vi "data_distributor.vi"(0 "Analog Data Array":T1[](array[typedef]), 7 "Refnums of Controls":T2[](array[typedef]), 9 "Indicies":T3[](array[typedef]), 11 "error in":errorcluster) -> (15 "error out":errorcluster)   [LabVIEW 2017]
uses:
  Utility Sub VIs/pressure_temp_mixture.ctl
  Utility Sub VIs/pulse_generator_data_charts.ctl
  Utility Sub VIs/pulse_generator_data.ctl
  Utility Sub VIs/diode_charts.ctl
  index_array_cluster.ctl
  refnum_array_cluster.ctl
  Utility Sub VIs/valve_pid_control.ctl
  Box/Annular Flow/Jason/LabVIEW 2017/Input Channel Lists/analog_data.ctl
panel:
  in  "PID Refnum":refnum<vi>
  in  "Diode ChartsRefnum":refnum<vi>
  in  "Measurements Data Refnum":refnum<vi>
  in  "PG Charts Refnum":refnum<vi>
  in  "Pressure/Temperature/Mixture Properties Refnum":refnum<vi>
  # "Pulse Gen"
  # "Test Section"
  # "Saturation\nPressure [Pa]"
  # "Saturation\nTemperature [C]"
  # "Pressure [Pa]"
  # "Temperature [C]"
  # "Liquid Tank"
  # "Separator"
  # "Liquid Inlet"
  # "Vapor Tank"
  # "Vapor Inlet"
  # "Test Section"
  # "Upper Dev Section"
  # "Lower Dev Section"
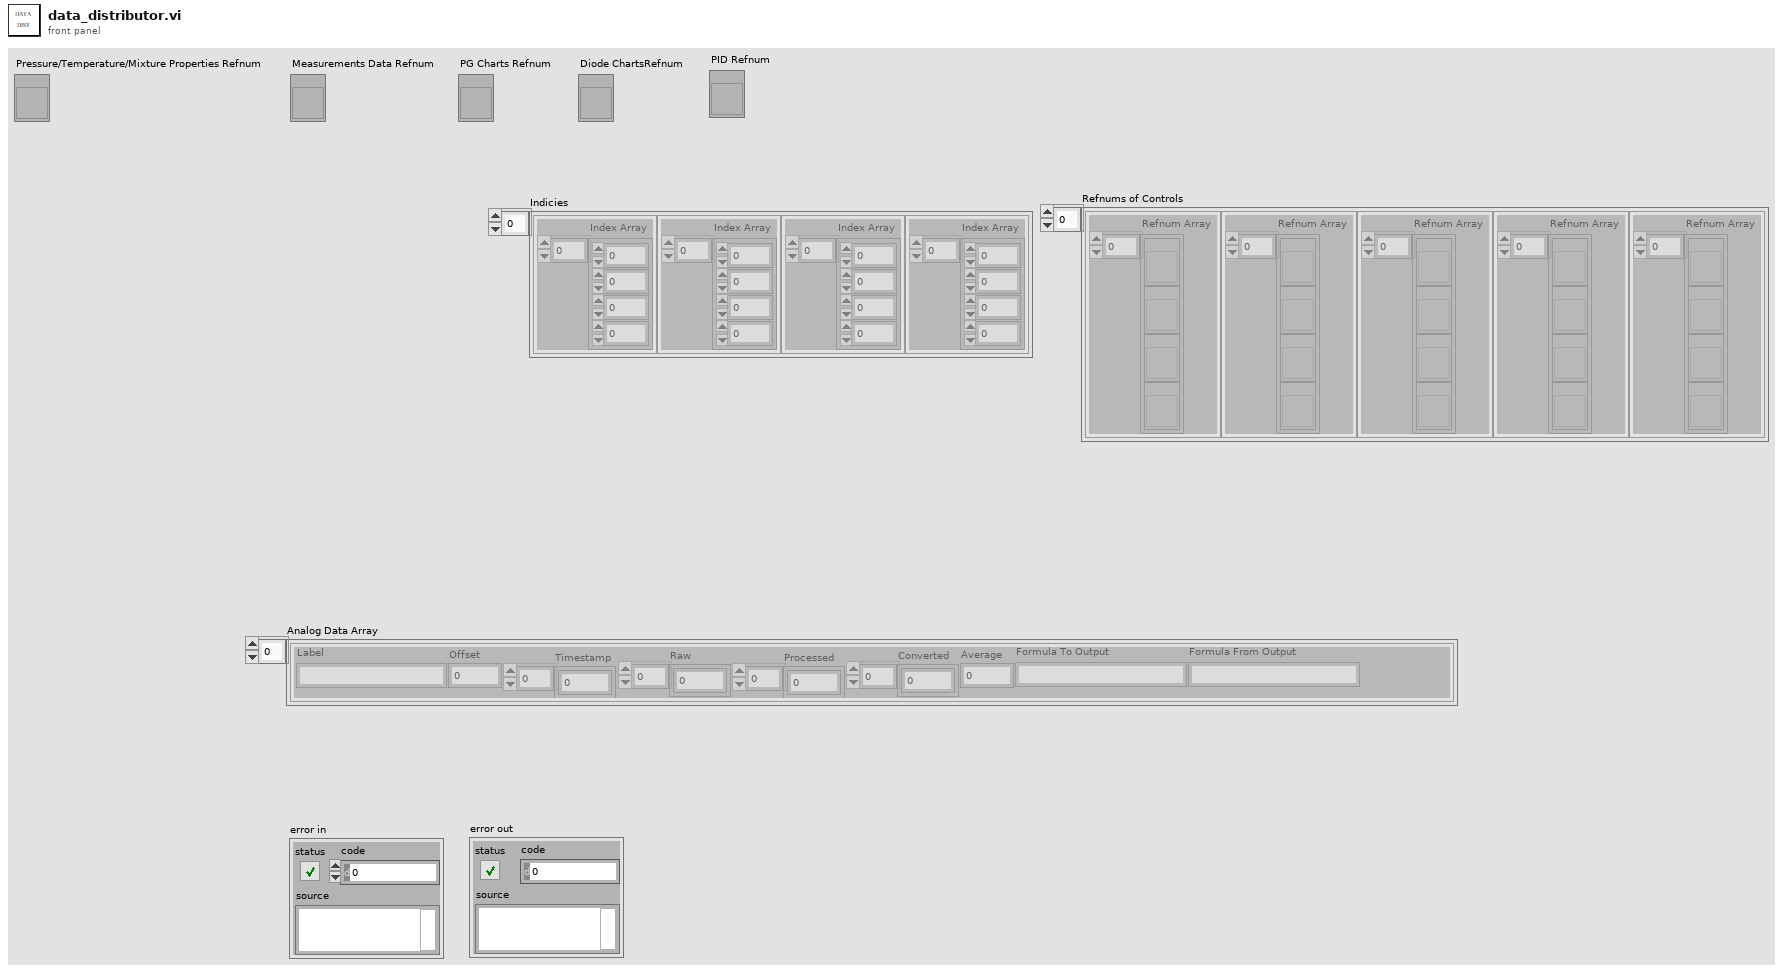
[diagram p1: front panel]
types:
  T1 = typedef "analog_data.ctl" = cluster{"Label":string, "Offset":dbl, "Timestamp":dbl[], "Raw":dbl[], "Processed":dbl[], "Converted":dbl[], "Average":dbl, "Formula To Output":string, "Formula From Output":string}
  T2 = typedef "refnum_array_cluster.ctl" = cluster{"Refnum Array":refnum<vi>[]}
  T3 = typedef "index_array_cluster.ctl" = cluster{"Index Array":i32[]}
  T4 = typedef "pressure_temp_mixture.ctl" = cluster{"Line Densities\n[g/cm^3]":cluster{"Vapor Line":dbl, "Liquid Line":dbl}, "Mixture Properties":cluster{"Enthalpy":dbl, "Quality [-]":dbl}, "Component PTs":cluster{"Liquid Tank P":dbl, "Liquid Tank T":dbl, "Liquid Tank Sat P":dbl, "Liquid Tank Sat T":dbl, "Separator P":dbl, "Separator T":dbl, "Separator Sat P":dbl, "Separator Sat T":dbl, "Liquid Inlet P":dbl, "Liquid Inlet T":dbl, "Liquid Inlet Sat P":dbl, "Liquid Inlet Sat T":dbl, "Vapor Tank P":dbl, "Vapor Tank T":dbl, "Vapor Tank Sat P":dbl, "Vapor Tank Sat T":dbl, "Vapor Inlet P":dbl, "Vapor Inlet T":dbl, "Vapor Inlet Sat P":dbl, "Vapor Inlet Sat T":dbl, "Test Section P":dbl, "Test Section T":dbl, "Test Section Sat P":dbl, "Test Section Sat T":dbl, "Upper Dev Section P":dbl, "Upper Dev Section T":dbl, "Upper Dev Section Sat P":dbl, "Upper Dev Section Sat T":dbl, "Lower Dev Section P":dbl, "Lower Dev Section T":dbl, "Lower Dev Section Sat P":dbl, "Lower Dev Section Sat T":dbl}, "Ambient Pressure [Pa]":dbl, "Mixing Tee":cluster{"Mixing Tee dP":dbl, "PG inlet-Mixing Tee Abs Pressure":dbl, "PG inlet-Mixing Tee Temperature":dbl}}
  T5 = cluster{"[0]":dbl, "[1]":dbl, "[2]":dbl, "[3]":dbl, "[4]":dbl, "[5]":dbl, "[6]":dbl, "[7]":dbl, "[8]":dbl, "[9]":dbl, "[10]":dbl, "[11]":dbl, "[12]":dbl, "[13]":dbl, "[14]":dbl, "[15]":dbl, "[16]":dbl, "[17]":dbl, "[18]":dbl, "[19]":dbl, "[20]":dbl, "[21]":dbl, "[22]":dbl, "[23]":dbl, "[24]":dbl, "[25]":dbl, "[26]":dbl, "[27]":dbl, "[28]":dbl, "[29]":dbl, "[30]":dbl, "[31]":dbl}
  T6 = cluster{"Mass Flow Rate [g/s]":dbl, "Mass Flow Rate [g/s]":dbl}
  T7 = cluster{"[0]":dbl, "[1]":dbl, "[2]":dbl, "[3]":dbl, "[4]":dbl, "[5]":dbl, "[6]":dbl, "[7]":dbl, "[8]":dbl, "[9]":dbl, "[10]":dbl, "[11]":dbl, "[12]":dbl, "[13]":dbl, "[14]":dbl, "[15]":dbl}
  T8 = typedef "valve_pid_control.ctl" = cluster{"proportional gain (Kc)":dbl, "integral time (Ti, min)":dbl, "derivative time (Td, min)":dbl, "Valve Voltage [V]":dbl, "Min % Open":dbl, "Max % Open":dbl, "Reinitialize?":bool, "Valve On/Off":bool, "Mode":bool, "Full Flow Rate":dbl, "Flow Set Point [g/s]":dbl, "AutoTune":bool, "Flow":cluster{"Flow rate [g/s]":dbl, "Line Density [g/cm^3]":dbl}}
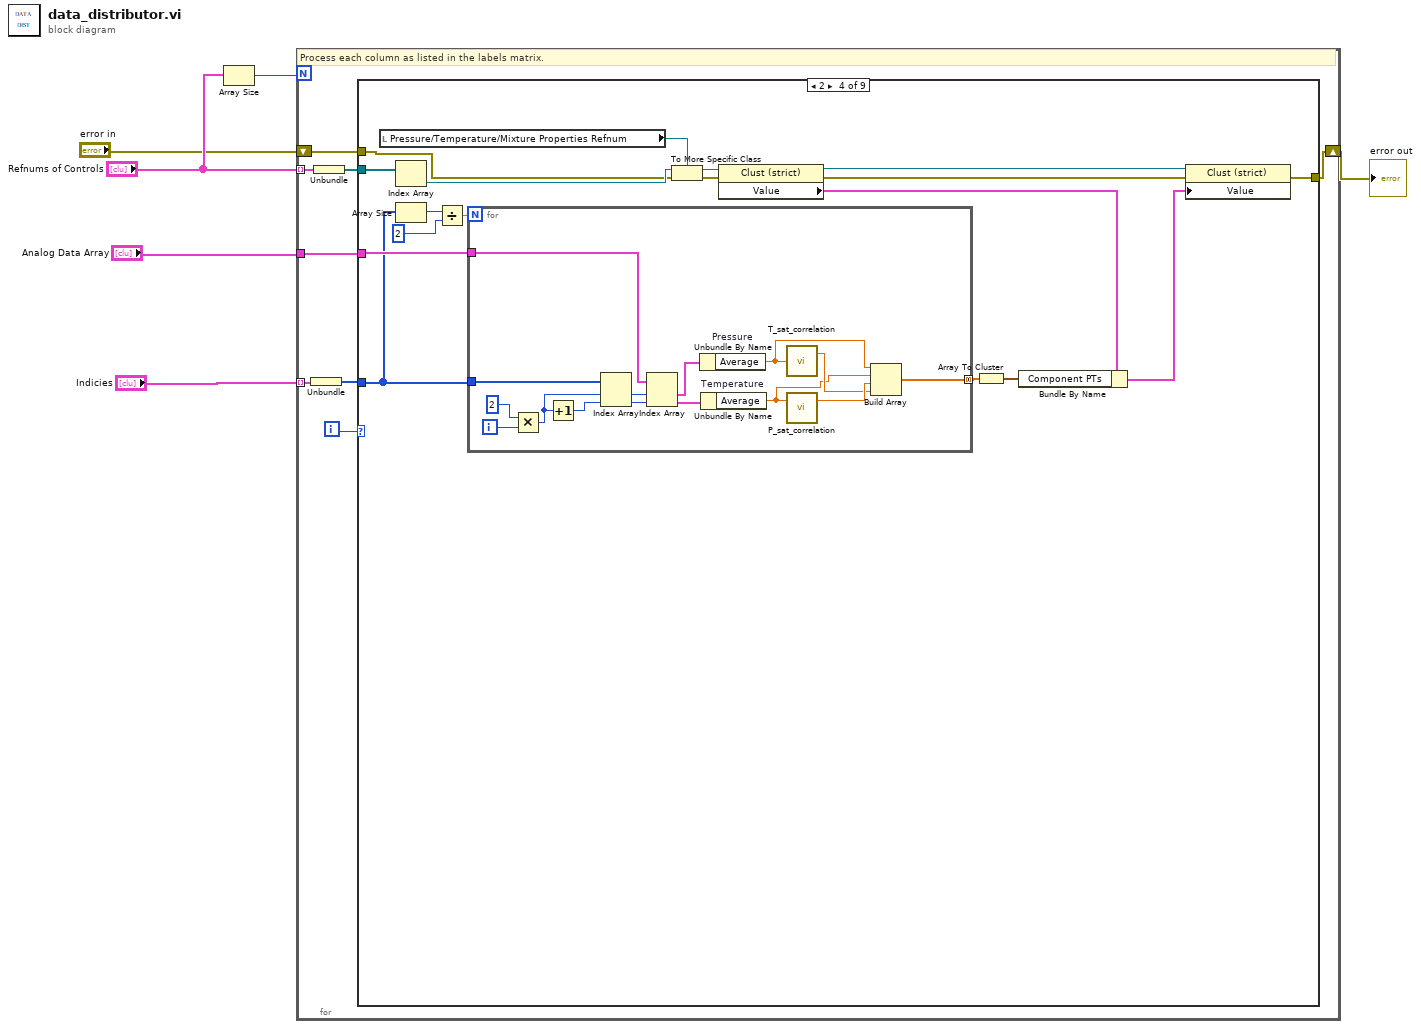
[diagram p0: block diagram]
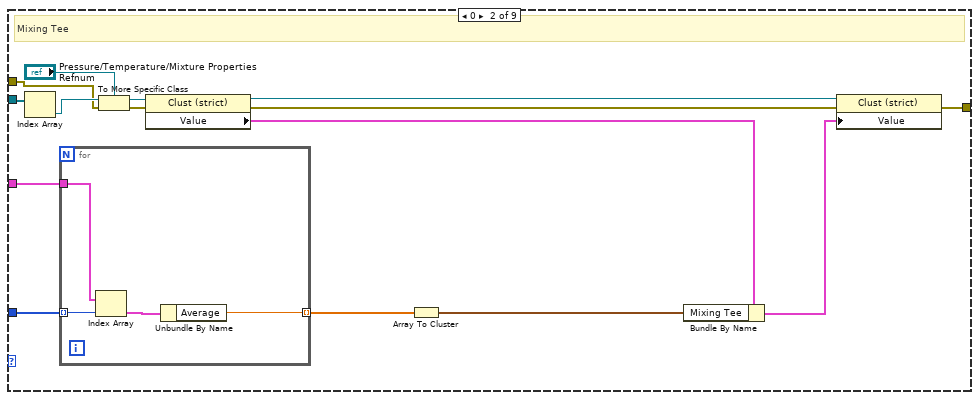
[diagram p3: hidden frame]
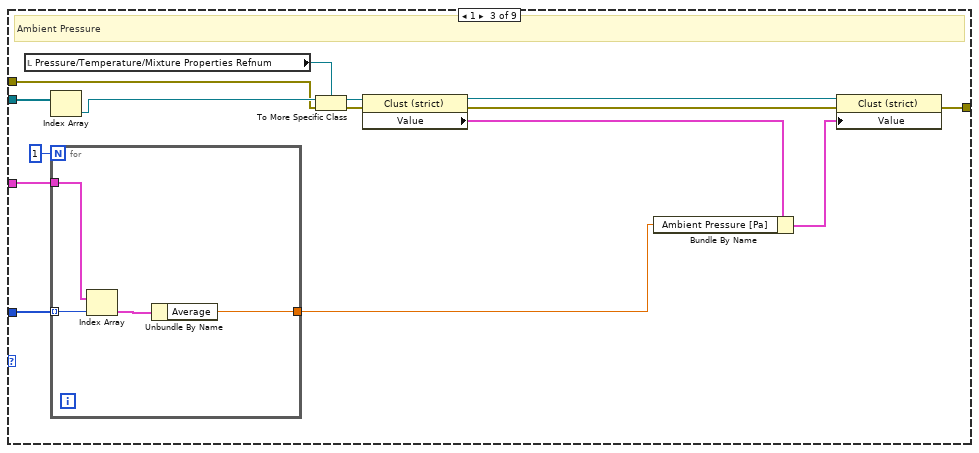
[diagram p4: hidden frame]
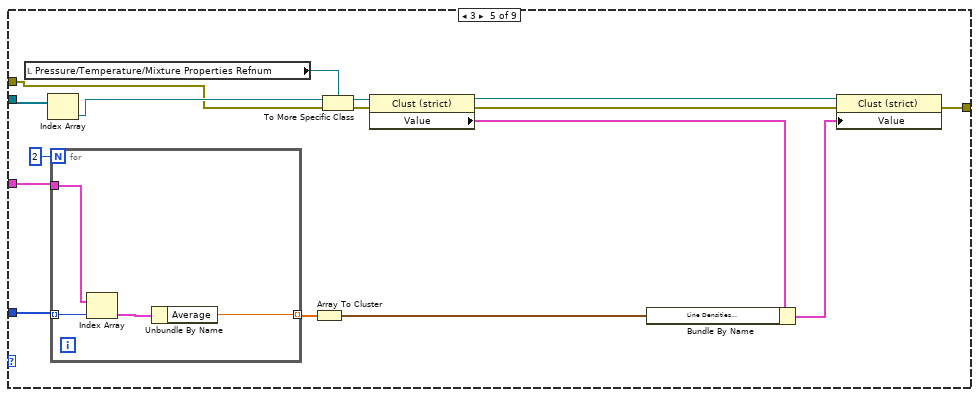
[diagram p5: hidden frame]
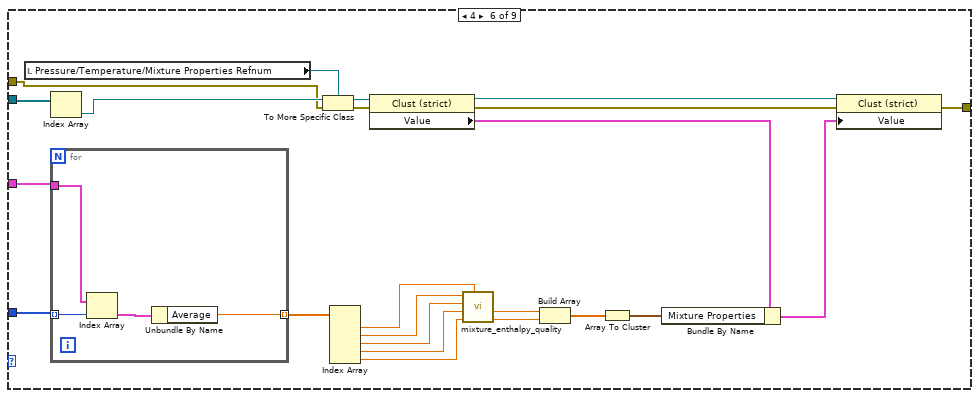
[diagram p6: hidden frame]
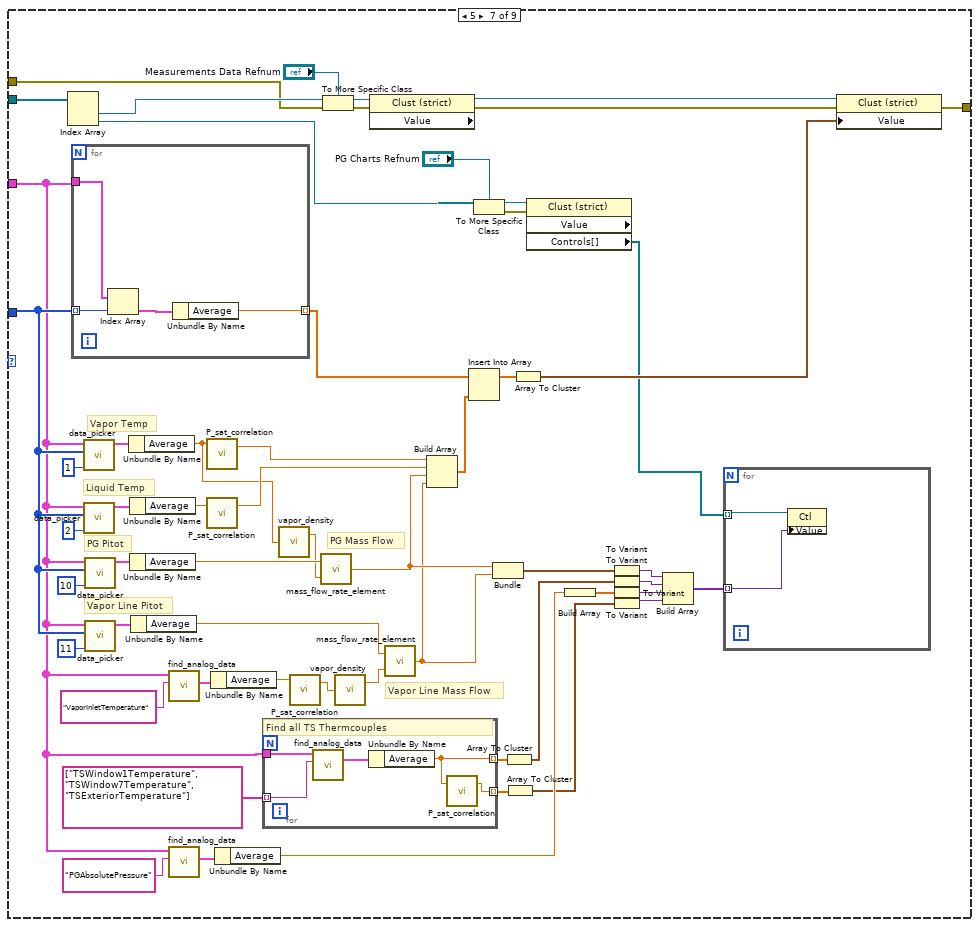
[diagram p7: hidden frame]
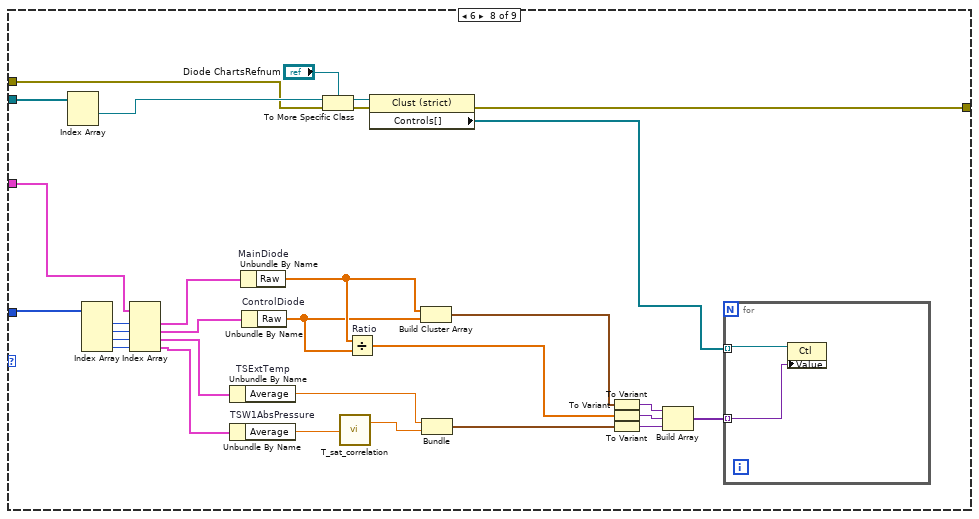
[diagram p8: hidden frame]
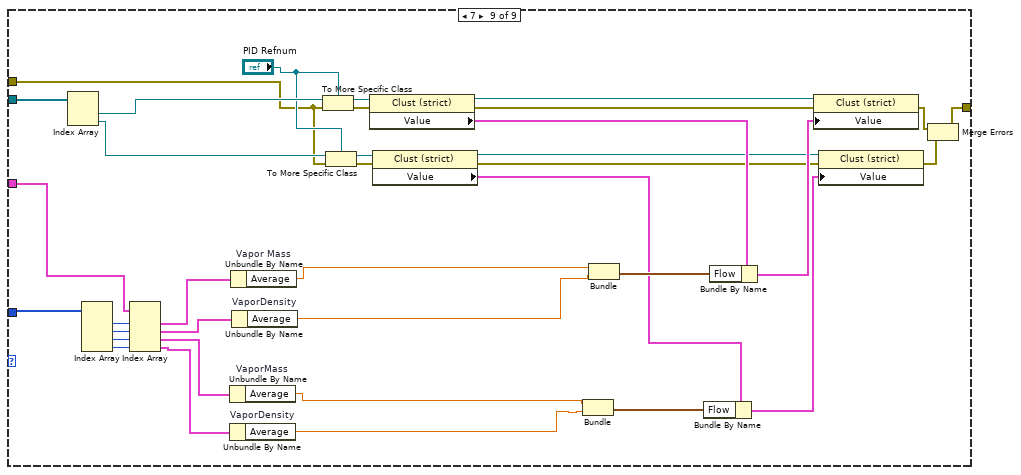
[diagram p9: hidden frame]
diagram:
  n1 = Array Size(array="Refnums of Controls") -> (size(s)=w3:i32)
  n2 = for {
    N: w3 -> [_]
    tunnel: "Analog Data Array" -> [w13]
    tunnel: "Indicies" -> [w10] mode=indexing
    tunnel: "Refnums of Controls" -> [w12] mode=indexing
    shift-right: [w7] -> w5
    shift-left: "error in" -> [w8]
    i -> [w14]
    # "Process each column as listed in the labels matrix."
    n3 = Unbundle(w10) -> ("Index Array"=w9:i32[])
    n4 = Unbundle(w12) -> ("Refnum Array"=w11:refnum<vi>[])
    n5 = case shown="2" w14 {
      tunnel: w9 -> [_ w23 w42 w63 w94 w121 w177 w221 w265]
      tunnel: w11 -> [_ w16 w38 w57 w90 w110 w147 w227 w266]
      tunnel: w13 -> [_ w22 w43 w64 w95 w122 w152 w219 w263]
      tunnel: w8 -> [w15 w18 w36 w55 w88 w108 w136 w203 w251]
      tunnel: [w15 w17 w35 w54 w87 w107 w135 w202 w234] -> w7
      frame Default {
      }
      frame 0 {
        # "Mixing Tee"
        n6 = Index Array(array=w16) -> (element=w19:refnum<vi>)  [unwired: 1 in]
        n7 = for {
          tunnel: w23 -> [w34] mode=indexing
          tunnel: w22 -> [w33]
          tunnel: [w31] -> w21 mode=indexing
          n8 = Index Array(array=w33, index=w34) -> (element=w32:T1)
          n9 = Unbundle By Name(w32) -> ("Average"=w31:dbl)
        }
        n10 = To More Specific Class(target class="Pressure/Temperature/Mixture Properties Refnum", reference=w19, error in=w18) -> (specific class reference=w29:refnum<vi>, error out=w28:errorcluster)
        n11 = property class="Clust (strict)"(reference=w29, error in=w28) -> (reference out=w24:refnum<vi>, error out=w25:errorcluster, "Value"=w27:T4)
        n12 = Array To Cluster(array=w21) -> (cluster=w20:cluster{"[0]":dbl, "[1]":dbl, "[2]":dbl})
        n13 = Bundle By Name(cluster=w27, "Mixing Tee"=w20) -> (w26:T4)
        n14 = property class="Clust (strict)"(reference=w24, error in=w25, "Value"=w26) -> (error out=w17:errorcluster)  [unwired: 1 out]
      }
      frame 1 {
        # "Ambient Pressure"
        n15 = local read "Pressure/Temperature/Mixture Properties Refnum"() -> (w40:refnum<vi>)
        n16 = Index Array(array=w38) -> (element=w37:refnum<vi>)  [unwired: 1 in]
        n17 = for {
          N: 1 -> [_]
          tunnel: w42 -> [w53] mode=indexing
          tunnel: w43 -> [w52]
          tunnel: [w50] -> w41
          n18 = Index Array(array=w52, index=w53) -> (element=w51:T1)
          n19 = Unbundle By Name(w51) -> ("Average"=w50:dbl)
        }
        n20 = To More Specific Class(target class=w40, reference=w37, error in=w36) -> (specific class reference=w49:refnum<vi>, error out=w48:errorcluster)
        n21 = property class="Clust (strict)"(reference=w49, error in=w48) -> (reference out=w44:refnum<vi>, error out=w45:errorcluster, "Value"=w47:T4)
        n22 = Bundle By Name(cluster=w47, "Ambient Pressure [Pa]"=w41) -> (w46:T4)
        n23 = property class="Clust (strict)"(reference=w44, error in=w45, "Value"=w46) -> (error out=w35:errorcluster)  [unwired: 1 out]
      }
      frame 2 {
        n24 = local read "Pressure/Temperature/Mixture Properties Refnum"() -> (w65:refnum<vi>)
        n25 = Index Array(array=w57) -> (element=w56:refnum<vi>)  [unwired: 1 in]
        n26 = Array Size(array=w63) -> (size(s)=w61:i32)
        n27 = Divide(x=w61, y=2) -> (x/y=w62:dbl)
        n28 = for {
          N: w62 -> [_]
          tunnel: w63 -> [w82]
          tunnel: w64 -> [w86]
          tunnel: [w72] -> w59 mode=concatenating
          i -> [w84]
          n29 = Multiply(x=2, y=w84) -> (x*y=w80:i32)
          n30 = Increment(x=w80) -> (x+1=w81:i32)
          n31 = Index Array(array=w82, index #1=w80, index #2=w81) -> (element #1=w79:i32, element #2=w78:i32)
          n32 = Index Array(array=w86, index #1=w79, index #2=w78) -> (element #1=w85:T1, element #2=w77:T1)
          n33 = Unbundle By Name "Pressure"(w85) -> ("Average"=w74:dbl)
          n34 = Unbundle By Name "Temperature"(w77) -> ("Average"=w73:dbl)
          n35 = call "T_sat_correlation.vi"("P [Pa]"=w74) -> ("T Sat [C]"=w75:dbl)  [unwired: 1 out]
          n36 = call "P_sat_correlation.vi"("Temperature[C]"=w73) -> ("P Sat[Pa]"=w76:dbl)  [unwired: 1 in, 1 out]
          n37 = Build Array(w74, w73, w76, w75) -> (w72:dbl[])
        }
        n38 = To More Specific Class(target class=w65, reference=w56, error in=w55) -> (specific class reference=w71:refnum<vi>, error out=w70:errorcluster)
        n39 = property class="Clust (strict)"(reference=w71, error in=w70) -> (reference out=w66:refnum<vi>, error out=w67:errorcluster, "Value"=w69:T4)
        n40 = Array To Cluster(array=w59) -> (cluster=w58:T5)
        n41 = Bundle By Name(cluster=w69, "Component PTs"=w58) -> (w68:T4)
        n42 = property class="Clust (strict)"(reference=w66, error in=w67, "Value"=w68) -> (error out=w54:errorcluster)  [unwired: 1 out]
      }
      frame 3 {
        n43 = local read "Pressure/Temperature/Mixture Properties Refnum"() -> (w96:refnum<vi>)
        n44 = Index Array(array=w90) -> (element=w89:refnum<vi>)  [unwired: 1 in]
        n45 = for {
          N: 2 -> [_]
          tunnel: w94 -> [w106] mode=indexing
          tunnel: w95 -> [w105]
          tunnel: [w103] -> w93 mode=indexing
          n46 = Index Array(array=w105, index=w106) -> (element=w104:T1)
          n47 = Unbundle By Name(w104) -> ("Average"=w103:dbl)
        }
        n48 = Array To Cluster(array=w93) -> (cluster=w92:cluster{"[0]":dbl, "[1]":dbl})
        n49 = To More Specific Class(target class=w96, reference=w89, error in=w88) -> (specific class reference=w102:refnum<vi>, error out=w101:errorcluster)
        n50 = property class="Clust (strict)"(reference=w102, error in=w101) -> (reference out=w97:refnum<vi>, error out=w98:errorcluster, "Value"=w100:T4)
        n51 = Bundle By Name(cluster=w100, "Line Densities\n[g/cm^3]"=w92) -> (w99:T4)
        n52 = property class="Clust (strict)"(reference=w97, error in=w98, "Value"=w99) -> (error out=w87:errorcluster)  [unwired: 1 out]
      }
      frame 4 {
        n53 = local read "Pressure/Temperature/Mixture Properties Refnum"() -> (w123:refnum<vi>)
        n54 = Index Array(array=w110) -> (element=w109:refnum<vi>)  [unwired: 1 in]
        n55 = for {
          tunnel: w121 -> [w133] mode=indexing
          tunnel: w122 -> [w132]
          tunnel: [w130] -> w120 mode=indexing
          n56 = Index Array(array=w132, index=w133) -> (element=w131:T1)
          n57 = Unbundle By Name(w131) -> ("Average"=w130:dbl)
        }
        n58 = To More Specific Class(target class=w123, reference=w109, error in=w108) -> (specific class reference=w129:refnum<vi>, error out=w128:errorcluster)
        n59 = Index Array(array=w120) -> (element #1=w115:dbl, element #2=w114:dbl, element #3=w113:dbl, element #4=w112:dbl, element #5=w111:dbl)  [unwired: 5 in]
        n60 = property class="Clust (strict)"(reference=w129, error in=w128) -> (reference out=w124:refnum<vi>, error out=w125:errorcluster, "Value"=w127:T4)
        n61 = call "mixture_enthalpy_quality.vi"("Vapor Inlet Pressure [Pa]"=w115, "Separator Temp [C]"=w111, "Liquid Inlet Temp [C]"=w112, "Vapor Flow Rate [g/s]"=w113, "Liquid Flow Rate [g/s]"=w114) -> ("Quality [-]"=w118:dbl, "mixture enthalpy"=w119:dbl)  [unwired: 2 out]
        n62 = Build Array(w119, w118) -> (w117:dbl[])
        n63 = Array To Cluster(array=w117) -> (cluster=w116:cluster{"[0]":dbl, "[1]":dbl})
        n64 = Bundle By Name(cluster=w127, "Mixture Properties"=w116) -> (w126:T4)
        n65 = property class="Clust (strict)"(reference=w124, error in=w125, "Value"=w126) -> (error out=w107:errorcluster)  [unwired: 1 out]
      }
      frame 5 {
        # "Vapor Line Mass Flow"
        # "PG Mass Flow"
        # "PG Pitot"
        # "Vapor Line Pitot"
        # "Liquid Temp"
        # "Vapor Temp"
        n66 = Index Array(array=w147) -> (element #1=w149:refnum<vi>, element #2=w148:refnum<vi>)  [unwired: 2 in]
        n67 = for {
          tunnel: w177 -> [w201] mode=indexing
          tunnel: w152 -> [w200]
          tunnel: [w198] -> w168 mode=indexing
          n68 = Index Array(array=w200, index=w201) -> (element=w199:T1)
          n69 = Unbundle By Name(w199) -> ("Average"=w198:dbl)
        }
        n70 = call "data_picker.vi"("index"=1, "Indicies"=w177, "Data in"=w152) -> ("Data Out"=w159:T1)  [unwired: 8 in]
        n71 = call "data_picker.vi"("index"=2, "Indicies"=w177, "Data in"=w152) -> ("Data Out"=w183:T1)  [unwired: 8 in]
        n72 = call "data_picker.vi"("index"=10, "Indicies"=w177, "Data in"=w152) -> ("Data Out"=w180:T1)  [unwired: 8 in]
        n73 = call "data_picker.vi"("index"=11, "Indicies"=w177, "Data in"=w152) -> ("Data Out"=w181:T1)  [unwired: 8 in]
        n74 = Unbundle By Name(w159) -> ("Average"=w134:dbl)
        n75 = Unbundle By Name(w183) -> ("Average"=w182:dbl)
        n76 = Unbundle By Name(w180) -> ("Average"=w176:dbl)
        n77 = Unbundle By Name(w181) -> ("Average"=w169:dbl)
        n78 = call "find_analog_data.vi"("Needle"="VaporInletTemperature", "Haystack"=w152) -> ("Needle Out"=w173:T1)  [unwired: 7 in, 2 out]
        n79 = call "find_analog_data.vi"("Needle"="PGAbsolutePressure", "Haystack"=w152) -> ("Needle Out"=w157:T1)  [unwired: 7 in, 2 out]
        n80 = call "P_sat_correlation.vi"("Temperature[C]"=w134) -> ("P Sat[Pa]"=w167:dbl)  [unwired: 1 in, 1 out]
        n81 = call "P_sat_correlation.vi"("Temperature[C]"=w182) -> ("P Sat[Pa]"=w166:dbl)  [unwired: 1 in, 1 out]
        n82 = Unbundle By Name(w173) -> ("Average"=w172:dbl)
        n83 = Unbundle By Name(w157) -> ("Average"=w156:dbl)
        n84 = for {
          tunnel: string[] ["TSWindow1Temperature", "TSWindow7Temperature", "TSExteriorTemperature"] ("Needle") -> [w196] mode=indexing
          tunnel: w152 -> [w197]
          tunnel: [w194] -> w151 mode=indexing
          tunnel: [w193] -> w150 mode=indexing
          # "Find all TS Thermcouples"
          n85 = call "find_analog_data.vi"("Needle"=w196, "Haystack"=w197) -> ("Needle Out"=w195:T1)  [unwired: 7 in, 2 out]
          n86 = Unbundle By Name(w195) -> ("Average"=w194:dbl)
          n87 = call "P_sat_correlation.vi"("Temperature[C]"=w194) -> ("P Sat[Pa]"=w193:dbl)  [unwired: 1 in, 1 out]
        }
        n88 = call "vapor_density.vi"("Vapor Temp [C]"=w134) -> ("Vapor Density[g/cm3]"=w175:dbl)  [unwired: 1 out]
        n89 = call "P_sat_correlation.vi"("Temperature[C]"=w172) -> ("P Sat[Pa]"=w171:dbl)  [unwired: 1 in, 1 out]
        n90 = call "mass_flow_rate_element.vi"("Density [g/cm3]"=w175, "dP [Pa]"=w176) -> ("Mass Flow Rate [g/s]"=w155:dbl)
        n91 = To More Specific Class(target class="Measurements Data Refnum", reference=w149, error in=w136) -> (specific class reference=w190:refnum<vi>, error out=w189:errorcluster)
        n92 = call "vapor_density.vi"("Vapor Temp [C]"=w171) -> ("Vapor Density[g/cm3]"=w170:dbl)  [unwired: 1 out]
        n93 = property class="Clust (strict)" props=["Value"](reference=w190, error in=w189) -> (reference out=w187:refnum<vi>, error out=w188:errorcluster)  [unwired: 1 out]
        n94 = call "mass_flow_rate_element.vi"("Density [g/cm3]"=w170, "dP [Pa]"=w169) -> ("Mass Flow Rate [g/s]"=w154:dbl)
        n95 = Build Array(w167, w166, w155, w154) -> (w165:dbl[])
        n96 = Insert Into Array(array=w168, new element=w165) -> (w164:dbl[])  [unwired: 1 in]
        n97 = To More Specific Class(target class="PG Charts Refnum", reference=w148) -> (specific class reference=w162:refnum<vi>, error out=w161:errorcluster)  [unwired: 1 in]
        n98 = Bundle("Mass Flow Rate [g/s]"=w155, "Mass Flow Rate [g/s]"=w154) -> (w145:T6)  [unwired: 1 in]
        n99 = Array To Cluster(array=w151) -> (cluster=w144:cluster{"[0]":dbl, "[1]":dbl, "[2]":dbl})
        n100 = Array To Cluster(array=w150) -> (cluster=w142:cluster{"[0]":dbl, "[1]":dbl})
        n101 = Array To Cluster(array=w164) -> (cluster=w163:T7)
        n102 = property class="Clust (strict)" props=["Value", "Controls[]"](reference=w162, error in=w161) -> ("Controls[]"=w146:refnum<vi>[])  [unwired: 3 out]
        n103 = Build Array(w156) -> (w143:dbl[])
        n104 = To Variant(anything=w145) -> (Variant=w141:variant)
        n105 = To Variant(anything=w144) -> (Variant=w140:variant)
        n106 = To Variant(anything=w143) -> (Variant=w139:variant)
        n107 = To Variant(anything=w142) -> (Variant=w138:variant)
        n108 = Build Array(w141, w140, w139, w138) -> (w137:variant[])
        n109 = for {
          tunnel: w146 -> [w192] mode=indexing
          tunnel: w137 -> [w191] mode=indexing
          n110 = property class="Ctl"(reference=w192, "Value"=w191) -> ()  [unwired: 1 in, 2 out]
        }
        n111 = property class="Clust (strict)"(reference=w187, error in=w188, "Value"=w163) -> (error out=w135:errorcluster)  [unwired: 1 out]
      }
      frame 6 {
        n112 = Index Array(array=w227) -> (element #1=w228:refnum<vi>)  [unwired: 2 in, 1 out]
        n113 = Index Array(array=w221) -> (element #1=w216:i32, element #2=w220:i32, element #3=w218:i32, element #4=w217:i32)  [unwired: 4 in]
        n114 = Index Array(array=w219, index #1=w216, index #2=w220, index #3=w218, index #4=w217) -> (element #1=w215:T1, element #2=w214:T1, element #3=w209:T1, element #4=w208:T1)
        n115 = Unbundle By Name "TSExtTemp"(w209) -> ("Average"=w206:dbl)
        n116 = Unbundle By Name "TSW1AbsPressure"(w208) -> ("Average"=w207:dbl)
        n117 = Unbundle By Name "MainDiode"(w215) -> ("Raw"=w213:dbl[])
        n118 = Unbundle By Name "ControlDiode"(w214) -> ("Raw"=w212:dbl[])
        n119 = To More Specific Class(target class="Diode ChartsRefnum", reference=w228, error in=w203) -> (specific class reference=w231:refnum<vi>, error out=w230:errorcluster)
        n120 = call "T_sat_correlation.vi"("P [Pa]"=w207) -> ("T Sat [C]"=w205:dbl)  [unwired: 1 out]
        n121 = Divide "Ratio"(x=w213, y=w212) -> (x/y=w210:dbl[])
        n122 = property class="Clust (strict)"(reference=w231, error in=w230) -> (error out=w202:errorcluster, "Controls[]"=w222:refnum<vi>[])  [unwired: 1 out]
        n123 = Build Cluster Array(w213, w212) -> (w211:cluster{dbl, dbl}[])
        n124 = Bundle("Average"=w206, "T Sat [C]"=w205) -> (w204:cluster{"Average":dbl, "T Sat [C]":dbl})  [unwired: 1 in]
        n125 = To Variant(anything=w211) -> (Variant=w226:variant)
        n126 = To Variant(anything=w210) -> (Variant=w225:variant)
        n127 = To Variant(anything=w204) -> (Variant=w224:variant)
        n128 = Build Array(w226, w225, w224) -> (w223:variant[])
        n129 = for {
          tunnel: w222 -> [w233] mode=indexing
          tunnel: w223 -> [w232] mode=indexing
          n130 = property class="Ctl"(reference=w233, "Value"=w232) -> ()  [unwired: 1 in, 2 out]
        }
      }
      frame 7 {
        n131 = Index Array(array=w266) -> (element #1=w267:refnum<vi>, element #2=w252:refnum<vi>)  [unwired: 2 in]
        n132 = Index Array(array=w265) -> (element #1=w260:i32, element #2=w264:i32, element #3=w262:i32, element #4=w261:i32)  [unwired: 4 in]
        n133 = Index Array(array=w263, index #1=w260, index #2=w264, index #3=w262, index #4=w261) -> (element #1=w259:T1, element #2=w258:T1, element #3=w257:T1, element #4=w256:T1)
        n134 = Unbundle By Name "VaporMass"(w257) -> ("Average"=w242:dbl)
        n135 = Unbundle By Name "VaporDensity"(w256) -> ("Average"=w241:dbl)
        n136 = Unbundle By Name "Vapor Mass"(w259) -> ("Average"=w249:dbl)
        n137 = Unbundle By Name "VaporDensity"(w258) -> ("Average"=w248:dbl)
        n138 = To More Specific Class(target class="PID Refnum", reference=w267, error in=w251) -> (specific class reference=w269:refnum<vi>, error out=w268:errorcluster)
        n139 = To More Specific Class(target class="PID Refnum", reference=w252, error in=w251) -> (specific class reference=w254:refnum<vi>, error out=w255:errorcluster)
        n140 = property class="Clust (strict)"(reference=w269, error in=w268) -> (reference out=w246:refnum<vi>, error out=w245:errorcluster, "Value"=w250:T8)
        n141 = property class="Clust (strict)"(reference=w254, error in=w255) -> (reference out=w240:refnum<vi>, error out=w239:errorcluster, "Value"=w238:T8)
        n142 = Bundle("Average"=w242, "Average"=w241) -> (w243:cluster{"Average":dbl, "Average":dbl})  [unwired: 1 in]
        n143 = Bundle("Average"=w249, "Average"=w248) -> (w247:cluster{"Average":dbl, "Average":dbl})  [unwired: 1 in]
        n144 = Bundle By Name(cluster=w238, "Flow"=w243) -> (w237:T8)
        n145 = Bundle By Name(cluster=w250, "Flow"=w247) -> (w244:T8)
        n146 = property class="Clust (strict)"(reference=w246, error in=w245, "Value"=w244) -> (error out=w236:errorcluster)  [unwired: 1 out]
        n147 = property class="Clust (strict)"(reference=w240, error in=w239, "Value"=w237) -> (error out=w235:errorcluster)  [unwired: 1 out]
        n148 = Merge Errors(w236, w235) -> (w234:errorcluster)
      }
    }
  }
  "error out" <- w5
